vi "GetAvailableSamples.vi"(8 "error in (no error)":errorcluster, 11 "FpgaRef5761 In":refnum<class "FpgaRef5761.lvclass">) -> (0 "error out":errorcluster, 2 "available":u32, 3 "FpgaRef5761 Out":refnum<class "FpgaRef5761.lvclass">)   [LabVIEW 2018, in "FpgaRef5761.lvclass"]
uses:
  FpgaRef5761.lvclass
  FpgaRef5761.lvclass/FpgaRef5761.ctl
  <vilib>/Utility/error.llb/Error Cluster From Error Code.vi
  <vilib>/rvi/errors/niLvFpgaAdjustHostInterfaceError.vi
  <vilib>/rvi/interface/nirviMethod/nirviMethod.xnode
  5761 FPGA ref.ctl
  <vilib>/FPGAPlugInAG/Dynamic/niLvFpga_ReadFifo_Dynamic.vi
  <vilib>/rvi/errors/niLvFpgaMergeErrorWithErrorCode.vi
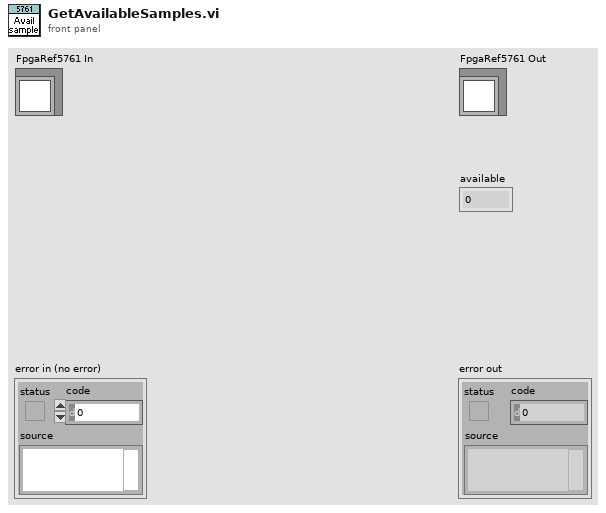
[diagram p1: front panel]
types:
  T1 = typedef "5761 FPGA ref.ctl" = refnum<k20>
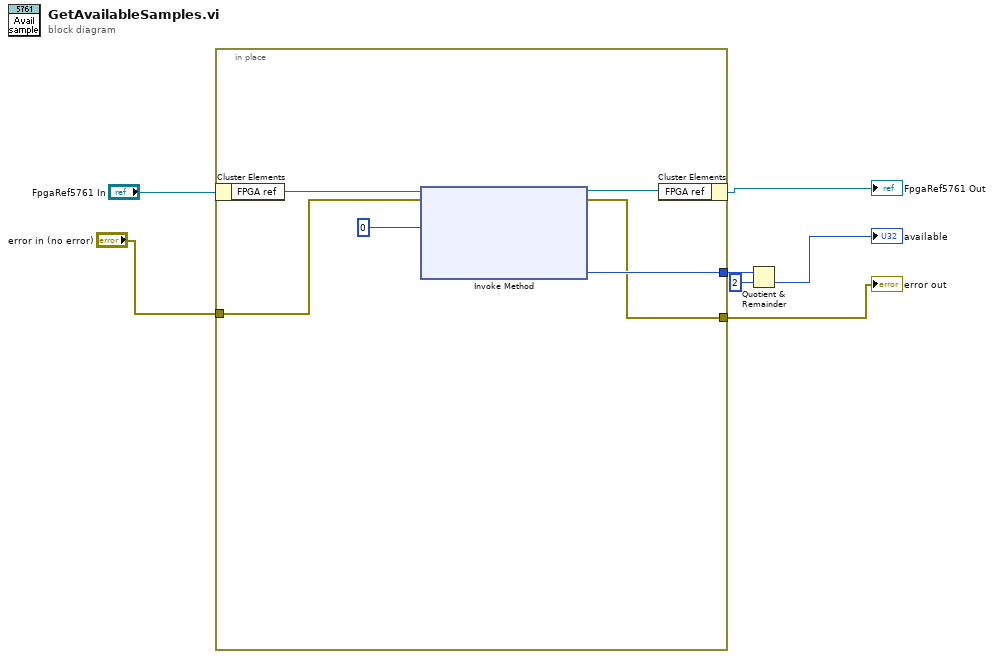
[diagram p0: block diagram]
diagram:
  n1 = in-place {
    in-place-border: [w10] -> w3
    in-place-border: "error in (no error)" -> [w9]
    in-place-border: [w8] -> w4
    n2 = in-place-cluster #1("FpgaRef5761 In") -> ("FPGA ref"=w12:T1)
    n3 = xnode "Invoke Method"("FPGA VI Reference In"=w12, "error in"=w9, "Number of Elements"=u32 0) -> ("FPGA VI Reference Out"=w11:T1, "error out"=w8:errorcluster, "Elements Remaining"=w10:u32)  [unwired: 1 in, 1 out]
    n4 = in-place-cluster #1("FPGA ref"=w11) -> (→"FpgaRef5761 Out":refnum<class "FpgaRef5761.lvclass">)
  }
  "error out" <- w4
  n5 = Quotient & Remainder(x=w3, y=u32 2) -> (floor(x/y)=→"available":u32)  [unwired: 1 out]
